vi "InitializeTF.vi"(9 "Image Path":path, 10 "Path to keras folder":path) -> (0 "error out":errorcluster, 3 "TFinfo out":T1)   [LabVIEW 2020]
panel:
  out "resulting string":string
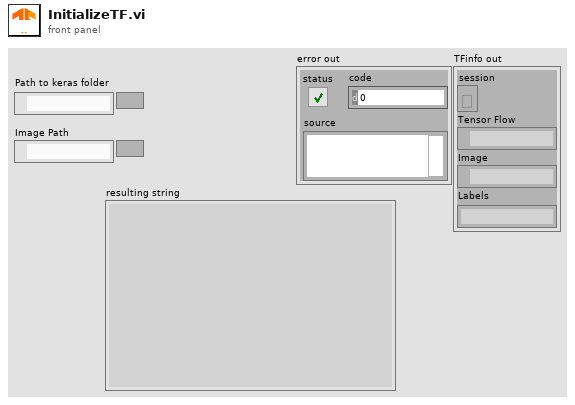
[diagram p1: front panel]
types:
  T1 = cluster{"session":refnum<k35>, "Tensor Flow":path, "Image":path, "Labels":string}
  T2 = cluster{"session out":refnum<k35>, "appended path":path, "Image Path":path, string}
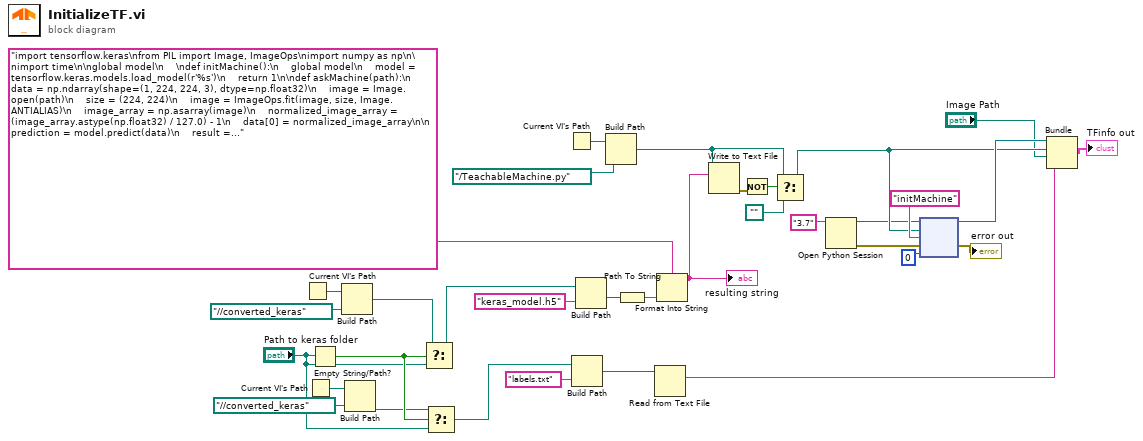
[diagram p0: block diagram]
diagram:
  n1 = Current VI's Path() -> (path=w21:path)
  n2 = Current VI's Path() -> (path=w17:path)
  n3 = Empty String/Path?(string/path="Path to keras folder") -> (empty?=w10:bool)
  n4 = Build Path(base path=w21, name or relative path=path "../../converted_keras") -> (appended path=w14:path)
  n5 = Build Path(base path=w17, name or relative path=path "../../converted_keras") -> (appended path=w9:path)
  n6 = Select(t=w14, s=w10, f="Path to keras folder") -> (s? t:f=w13:path)
  n7 = Select(t=w9, s=w10, f="Path to keras folder") -> (s? t:f=w7:path)
  n8 = Current VI's Path() -> (path=w27:path)
  n9 = Build Path(base path=w7, name or relative path="labels.txt") -> (appended path=w5:path)
  n10 = Build Path(base path=w13, name or relative path="keras_model.h5") -> (appended path=w11:path)
  n11 = Build Path(base path=w27, name or relative path=path "../TeachableMachine.py") -> (appended path=w25:path)
  n12 = Path To String(path=w11) -> (string=w19:string)
  n13 = Read from Text File(file (use dialog)=w5) -> (text=w15:string)  [unwired: 3 in, 3 out]
  n14 = Format Into String(format string="import tensorflow.keras\nfrom PIL import Image, ImageOps\nimport numpy as np\n\nimport time\n\nglobal model\n    \ndef initMachine():\n    global model\n    model = tensorflow.keras.models.load_model(r'%s')\n    return 1\n\ndef askMachine(path):\n    data = np.ndarray(shape=(1, 224, 224, 3), dtype=np.float32)\n    image = Image.open(path)\n    size = (224, 224)\n    image = ImageOps.fit(image, size, Image.ANTIALIAS)\n    image_array = np.asarray(image)\n    normalized_image_array = (image_array.astype(np.float32) / 127.0) - 1\n    data[0] = normalized_image_array\n\n    prediction = model.predict(data)\n    result = prediction.tolist()\n    return result\n" ("name or relative path"), w19) -> (resulting string=w18:string)  [unwired: 2 in, 1 out]
  "resulting string" <- w18
  n15 = Write to Text File(file (use dialog)=w25, text=w18) -> (error out=w33:errorcluster)  [unwired: 2 in, 2 out]
  n16 = Not(x=w33) -> (.not. x?=w31:bool)
  n17 = Select(t=w25, s=w31, f=path "") -> (s? t:f=w23:path)
  n18 = Open Python Session(python version="3.7" ("Python version")) -> (session out=w4:refnum<k35>, error out=w3:errorcluster)  [unwired: 2 in]
  n19 = node(w4, w23, "initMachine" ("function name"), w3, u8 0) -> (w24:refnum<k35>, →"error out":errorcluster)  [unwired: 1 in, 2 out]
  n20 = Bundle("session out"=w24, "appended path"=w23, "Image Path"="Image Path", w15) -> (→"TFinfo out":T2)  [unwired: 1 in]
